vi "程序设置-修改注释.vi"() -> (2 "程序号输出":i32, 3 "Cancelled?":bool caption="取消？")   [LabVIEW 2014]
doc: "该模板用于创建能够进行事件处理的对话框。"
panel:
  out "error out":errorcluster
  in  "错误输入":errorcluster caption="错误输入（无错误）"
  in  "程序注释":string
  in  "™C·Nßx“ñ":i32(ring) items=["程序0-----000"]
  in  "Cancel":bool caption="取消"
  in  "OK":bool caption="确定"
  # "修改程序注释"
  # "选中要修改\n的程序注释："
  # "修改程序注释："
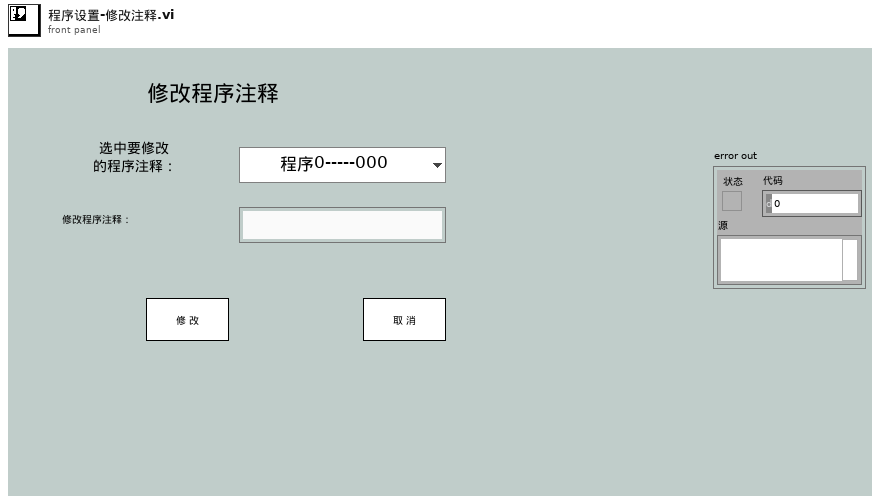
[diagram p1: front panel]
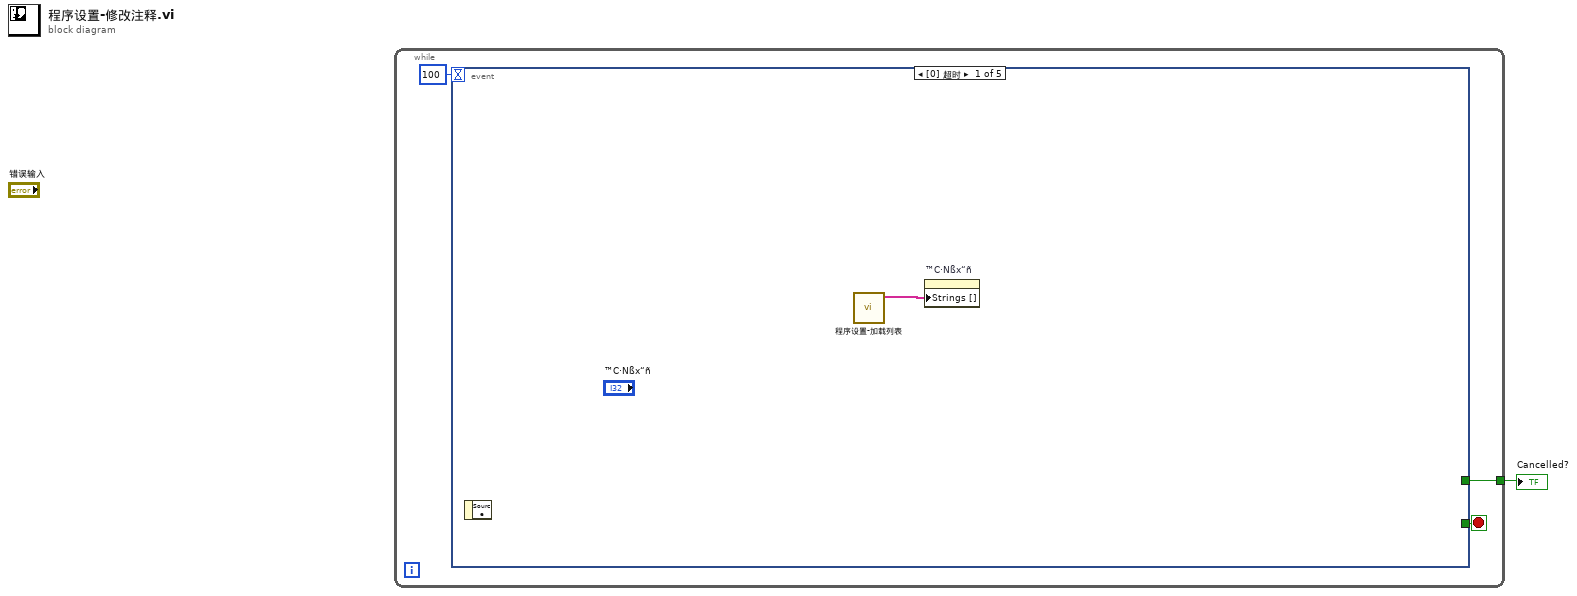
[diagram p0: block diagram]
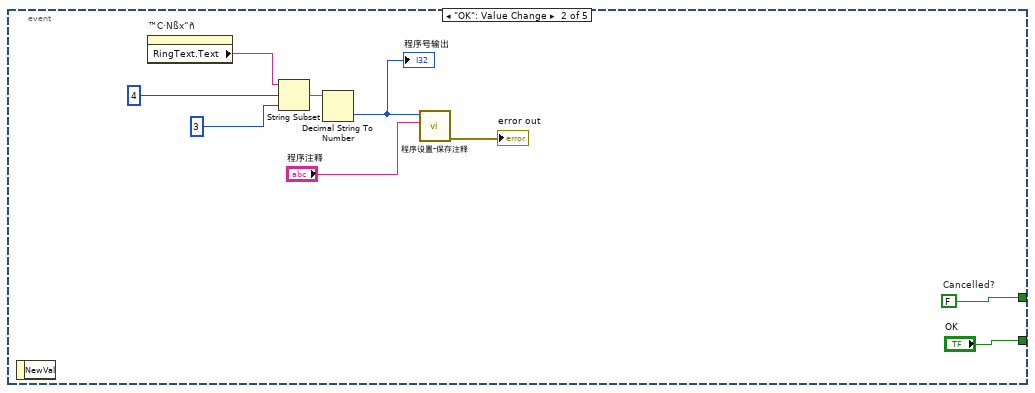
[diagram p2: hidden frame]
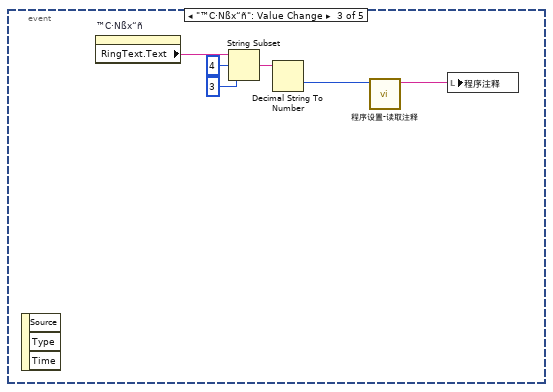
[diagram p3: hidden frame]
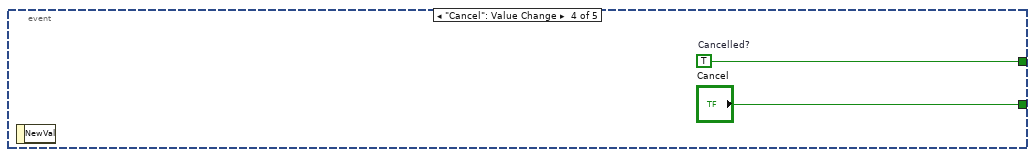
[diagram p4: hidden frame]
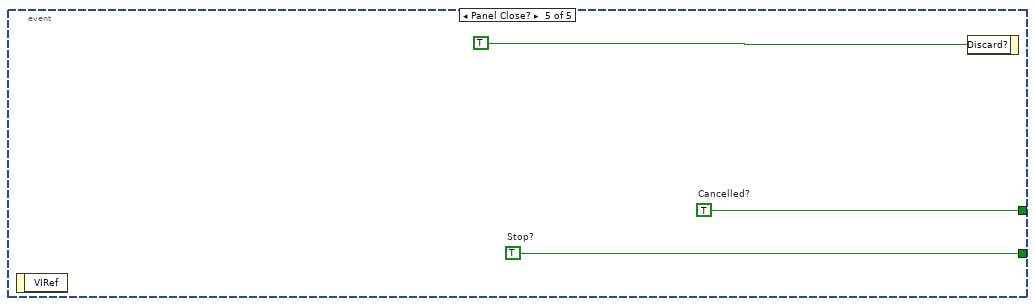
[diagram p5: hidden frame]
diagram:
  n1 = while {
    tunnel: [w3] -> w1
    stop <- w4 stop-if-true
    n2 = event shown="[0] 超时" {
      selector: _ -> [_ _ _ _ _]
      dyn-events: _ -> [_ _ _ _ _]
      timeout: 100 -> [_ _ _ _ _]
      tunnel: [_ "OK" _ "Cancel" w24] -> w4
      tunnel: [_ w14 _ w22 w23] -> w3
      event Timeout {
        n3 = event-data() -> ()  [unwired: 1 in, 1 out]
        n4 = call "程序设置-加载列表.vi"() -> ("文件名显示"=w5:string[])  [unwired: 10 in, 1 out]
        n5 = property on="™C·Nßx“ñ" class="Ring (严格)"("Strings []"=w5) -> ()  [unwired: 2 in, 2 out]
      }
      event "OK": Value Change {
        w14 = FALSE  # Cancelled?
        n6 = event-data() -> ()  [unwired: 1 in, 1 out]
        n7 = property on="™C·Nßx“ñ" class="Ring (严格)"() -> ("RingText.Text"=w7:string)  [unwired: 2 in, 2 out]
        n8 = String Subset(string=w7, offset (0)=4 ("偏移量(0)"), length (rest)=3 ("长度（剩余）")) -> (substring=w8:string)
        n9 = Decimal String To Number(string=w8) -> (number=w6:i32)  [unwired: 2 in, 1 out]
        "程序号输出" <- w6
        n10 = call "程序设置-保存注释.vi"("程序注释"="程序注释", "程序号"=w6) -> ("error out"=→"error out":errorcluster)  [unwired: 9 in]
      }
      event "™C·Nßx“ñ": Value Change {
        n11 = event-data() -> ()  [unwired: 1 in, 3 out]
        n12 = property on="™C·Nßx“ñ" class="Ring (严格)"() -> ("RingText.Text"=w20:string)  [unwired: 2 in, 2 out]
        n13 = String Subset(string=w20, offset (0)=4 ("偏移量(0)"), length (rest)=3 ("长度（剩余）")) -> (substring=w17:string)
        n14 = Decimal String To Number(string=w17) -> (number=w15:i32)  [unwired: 2 in, 1 out]
        n15 = call "程序设置-读取注释.vi"("程序号"=w15) -> ("程序注释"=w16:string)  [unwired: 9 in, 1 out]
        n16 = local write "程序注释"(w16) -> ()
      }
      event "Cancel": Value Change {
        w22 = TRUE  # Cancelled?
        n17 = event-data() -> ()  [unwired: 1 in, 1 out]
      }
      event Panel Close? {
        w23 = TRUE  # Cancelled?
        w24 = TRUE  # Stop?
        n18 = event-data() -> ()  [unwired: 1 in, 1 out]
        n19 = event-data("Discard?"=TRUE) -> ()  [unwired: 1 in, 1 out]
      }
    }
  }
  "Cancelled?" <- w1
